vi "GlobalShooter.vi"() -> ()   [LabVIEW 2023]
panel:
  out "SEN_Shooter_Upper_Temp(C)":dbl
  out "SEN_Shooter_Fault":bool[](array[boolean])
  out "SEN_Shooter_Overheating":bool[](array[boolean])
  out "OUT_Wrist_Stowed":bool
  out "SEN_Shooter_Rotator_Angle_(deg)":dbl
  out "OUT_Shooter_Firing":bool
  out "OUT_Shooter_Spinning":bool
  out "SEN_Shooter_Lower_Temp(C)":dbl
  out "SEN_Shooter_Upper_Velocity_(RPM)":dbl
  out "OUT_Shooter_Wrist":dbl
  out "REF_Shooter_Wrist":string
  out "OUT_Shooter_Diverter":bool
  out "REF_Shooter_Diverter":string
  out "REF_Shooter_Lower":string
  out "OUT_Shooter_Lower":dbl
  out "OUT_Shooter_Upper":dbl
  out "REF_Shooter_Upper":string
  # "DEVICE REFERENCE NAMES"
  # "OUTPUTS"
  # "Sensors"
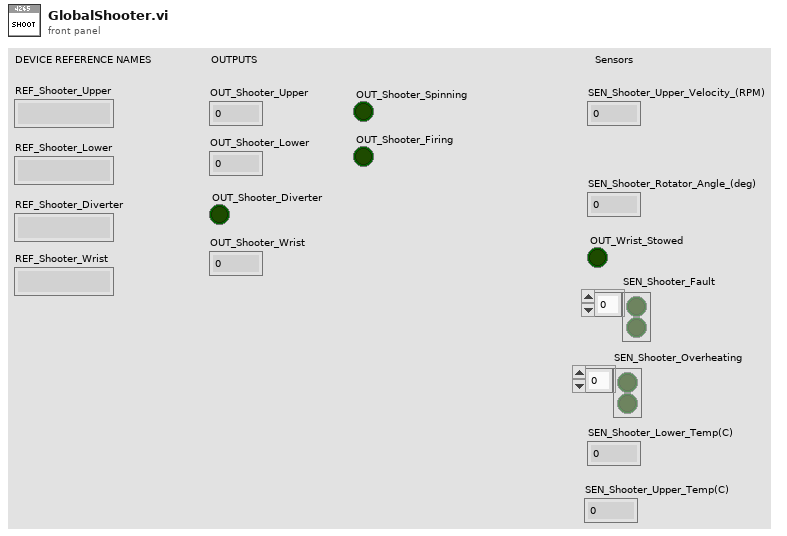
[diagram p1: front panel]
diagram:
